vi "Serial Example.vi"() -> ()   [LabVIEW 2023]
panel:
  in  "height":dbl
  in  "age":dbl
  in  "Gender":enum32{"Male", "Female"}(radio)
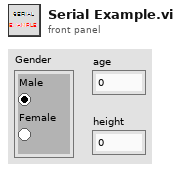
[diagram p1: front panel]
types:
  T1 = enum16{"Open", "Write Only", "Read Only", "Write&Read", "Close"}
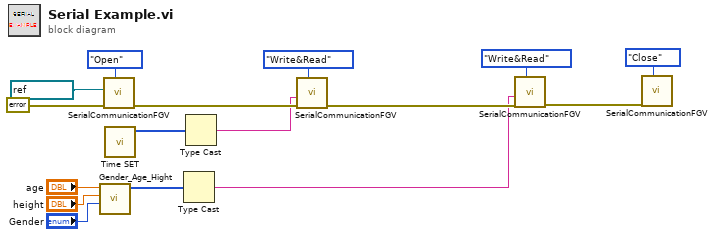
[diagram p0: block diagram]
diagram:
  n1 = call "Gender_Age_Hight.vi"("Gender"="Gender", "height"="height", "age"="age") -> ("Dataset"=w4:i32[])  [unwired: 8 in]
  n2 = call "SerialCommunicationFGV.vi"("ctl"=T1."Open", "errorIn"=errorcluster {"status"=FALSE, "code"=0, "source"=""}, "visaResourceNameIn"=refnum<visa-resource-name> "COM8") -> ("errorOut"=w13:errorcluster)  [unwired: 6 in, 2 out]
  n3 = call "Time SET.vi"() -> ("배열"=w6:i32[])  [unwired: 10 in, 1 out]
  n4 = Type Cast(x=w4) -> (*(type *) &x=w3:string)  [unwired: 1 in]
  n5 = Type Cast(x=w6) -> (*(type *) &x=w5:string)  [unwired: 1 in]
  n6 = call "SerialCommunicationFGV.vi"("ctl"=T1."Write&Read", "errorIn"=w13, "bufferWrite"=w5) -> ("errorOut"=w11:errorcluster)  [unwired: 6 in, 2 out]
  n7 = call "SerialCommunicationFGV.vi"("ctl"=T1."Write&Read", "errorIn"=w11, "bufferWrite"=w3) -> ("errorOut"=w1:errorcluster)  [unwired: 6 in, 2 out]
  n8 = call "SerialCommunicationFGV.vi"("ctl"=T1."Close", "errorIn"=w1) -> ()  [unwired: 7 in, 3 out]
